vi "ForwardToTarget.vi"   [LabVIEW 2016, in "Project 2 LabVIEW.lvrbt"]
uses:
  Project 2 LabVIEW.lvrbt
  <vilib>/NXT/Block Support/NXT_OutputPort.ctl
  <vilib>/NXT/Dual Mode Library/Waits/Wait_Num.vi
  <vilib>/NXT/NXTIO Xnodes/NXTIONodeSubVIs/NXTMoveMotors.vi
  <vilib>/NXT/NXTIO Xnodes/AddressXNode/NXTIOAddress.xnode
  <vilib>/NXT/NXTIO Xnodes/NXTIOXNode/NXTIO.xnode
  <vilib>/NXT/Subs/LVHSConnector.ctl
  <vilib>/NXT/LegoClasses/BrickReference/BrickReference.lvclass
types:
  T1 = typedef "NXT_OutputPort.ctl" = u8
  T2 = typedef "LVHSConnector.ctl" = refnum<class "BrickReference.lvclass">
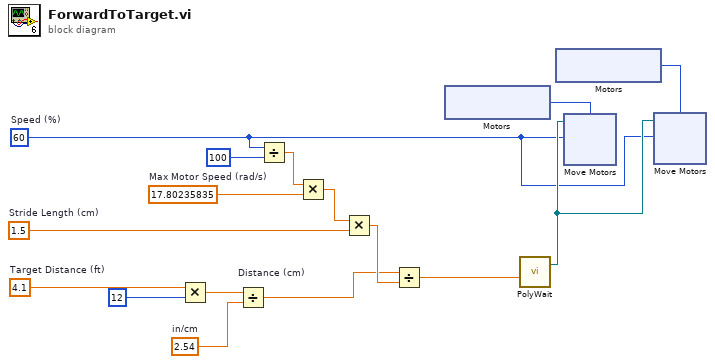
[diagram p0: block diagram]
diagram:
  w4 = 1.5  # Stride Length (cm)
  w6 = 17.80235835  # Max Motor Speed (rad/s)
  w10 = 2.54  # in/cm
  w9 = 60  # Speed (%)
  w13 = 4.1  # Target Distance (ft)
  n1 = Multiply(x=w13, y=12) -> (x*y=w11:dbl)
  n2 = Divide "Distance (cm)"(x=w11, y=w10) -> (x/y=w2:dbl)
  n3 = Divide(x=w9, y=100) -> (x/y=w7:dbl)
  n4 = Multiply(x=w7, y=w6) -> (x*y=w5:dbl)
  n5 = Multiply(x=w5, y=w4) -> (x*y=w3:dbl)
  n6 = Divide(x=w2, y=w3) -> (x/y=w1:dbl)
  n7 = xnode "Motors"() -> ("Motor"=w16:T1)
  n8 = call-poly <vilib>:"PolyWait.vi"("Time (1 sec)"=w1) -> ("NXT/EV3"=w14:T2)  [unwired: 3 in]
  n9 = xnode "Motors"() -> ("Motor"=w15:T1)
  n10 = xnode "Move Motors"("Power/Speed 1"=w9, "Motors"=w16, "NXT/EV3"=w14) -> ()  [unwired: 1 out]
  n11 = xnode "Move Motors"("Power/Speed 1"=w9, "Motors"=w15, "NXT/EV3"=w14) -> ()  [unwired: 1 out]
